vi "Destroy.vi"(8 "error in (no error)":errorcluster, 11 "Ring Buffer":T1) -> (0 "error out":errorcluster)   [LabVIEW 2021, in "Ring Buffer Strict Accessor.lvlib"]
uses:
  Ring Buffer Strict Accessor.lvlib
  SubVIs/RingBufferHandle.ctl
  <userlib>/bjustice/Ring Buffer for Time Series Data/SubVIs/DVR data.ctl
  SubVIs/DataType.ctl
  SubVIs/Endianess.ctl
  <userlib>/bjustice/Ring Buffer for Time Series Data/Ring Buffer Time Series Data.lvlib
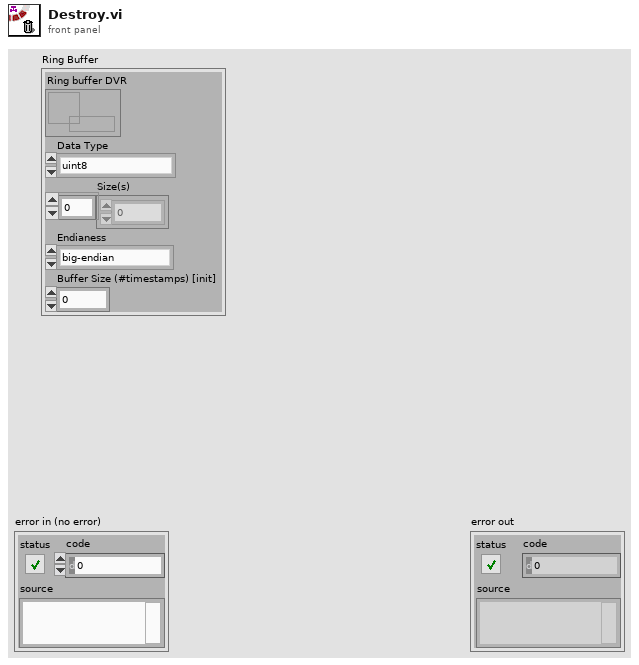
[diagram p1: front panel]
types:
  T1 = typedef "Ring Buffer Strict Accessor.lvlib/RingBufferHandle.ctl" = cluster{"Ring buffer DVR":refnum<data-value>, "Data Type":T2, "Size(s)":i32[], "Endianess":T3, "Buffer Size (#timestamps) [init]":i32}
  T2 = typedef "Ring Buffer Strict Accessor.lvlib/DataType.ctl" = enum16{"uint8", "uint16", "uint32", "uint64", "int8", "int16", "int32", "int64", "float", "double", "extended"}
  T3 = typedef "Ring Buffer Strict Accessor.lvlib/Endianess.ctl" = enum16{"big-endian", "little-endian"}
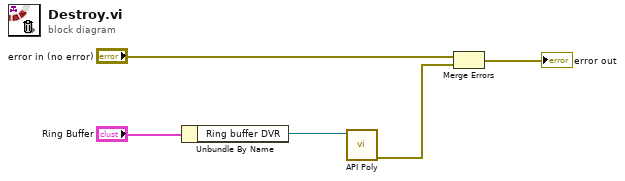
[diagram p0: block diagram]
diagram:
  n1 = Unbundle By Name("Ring Buffer") -> ("Ring buffer DVR"=w4:refnum<data-value>)
  n2 = call-poly <userlib>:"API Poly.vi"("Ring buffer DVR"=w4) -> ("error out"=w2:errorcluster)  [unwired: 10 in]
  n3 = Merge Errors("error in (no error)", w2) -> (→"error out":errorcluster)
